vi "MeasurementItems_SetTransferNumber.vi"(8 "error in (no error)":errorcluster, 10 "Num of items transfered (-1 for all)":i32, 11 "OXY_SCPI Reseource In":refnum<visa-resource-name>) -> (0 "error out":errorcluster, 1 "communication_data":T1, 3 "OXY_SCPI Reseource Out":refnum<visa-resource-name>)   [LabVIEW 2018, in "OXYGEN.lvlib"]
doc: "Sets the number of items to be transferred beginning from index 0"
uses:
  OXYGEN.lvlib
  TypeDefs/Cluster_RawCommData.ctl
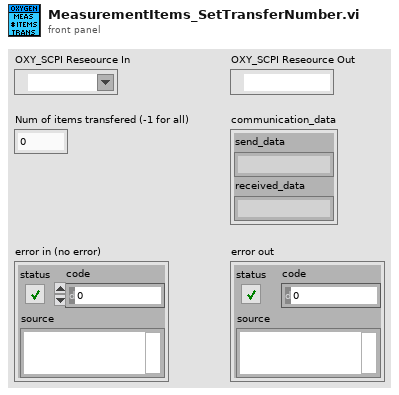
[diagram p1: front panel]
types:
  T1 = typedef "OXYGEN.lvlib/Cluster_RawCommData.ctl" = cluster{"send_data":string, "received_data":string}
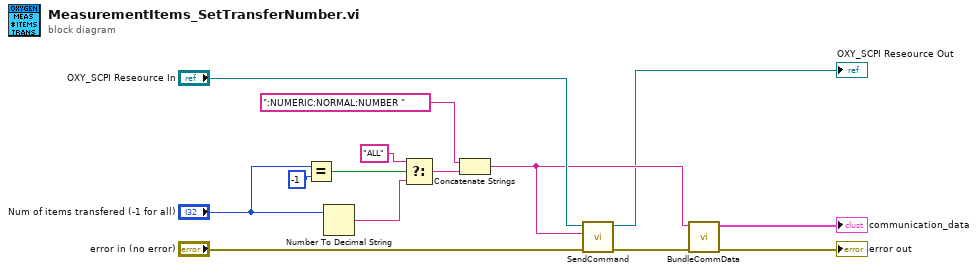
[diagram p0: block diagram]
diagram:
  n1 = Equal?(x="Num of items transfered (-1 for all)", y=-1) -> (x = y?=w9:bool)
  n2 = Number To Decimal String(number="Num of items transfered (-1 for all)") -> (decimal integer string=w1:string)  [unwired: 1 in]
  n3 = Select(t="ALL", s=w9, f=w1) -> (s? t:f=w6:string)
  n4 = Concatenate Strings(":NUMERIC:NORMAL:NUMBER " ("t"), w6) -> (w5:string)
  n5 = call "SendCommand.vi"("error in (no error)"="error in (no error)", "String to Send"=w5, "OXY_SCPI Reseource In"="OXY_SCPI Reseource In") -> ("error out"=w4:errorcluster, "OXY_SCPI Reseource Out"=→"OXY_SCPI Reseource Out":refnum<visa-resource-name>)  [unwired: 7 in]
  n6 = call "BundleCommData.vi"("error in (no error)"=w4, "send_data"=w5) -> ("error out"=→"error out":errorcluster, "communication_data"=→"communication_data":T1)  [unwired: 8 in]
